vi "Query Active DUT Band Restrictions.vi"(8 "error in (no error)":errorcluster, 9 "Band Number (1)":i32=1, 10 "Band Type (LTE)":i32(ring) items=["LTE", "New Radio"], 11 "VISA resource name":refnum<visa-resource-name>) -> (0 "error out":errorcluster, 1 "RX":i32, 2 "TX":i32, 3 "VISA resource name out":refnum<visa-resource-name>)   [LabVIEW 2020, in "Rohde&Schwarz CMXP Base.lvlib"]
doc: "Queries restrictions for a frequency band assigned to connectors of the active DUT.\n\nAttribute:\n-\n\nRemote-control command:\n[CONFigure:]DUT:BAND:RESTrictions"
uses:
  <instrlib>/Rohde&Schwarz CMXP Base/Rohde&Schwarz CMXP Base.lvlib
  <instrlib>/Rohde&Schwarz CMXP Base/Private/rsidr_core.llb/rsidr_core.lvlib
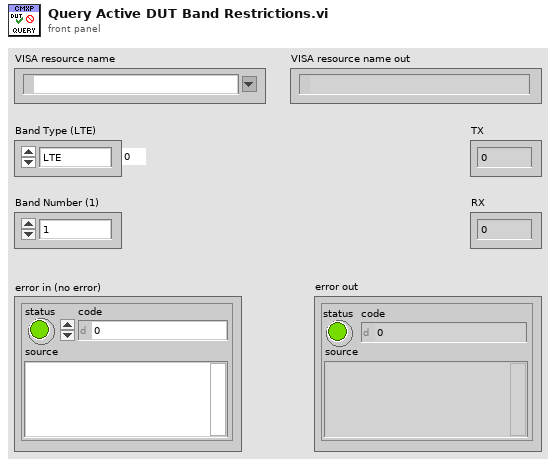
[diagram p1: front panel]
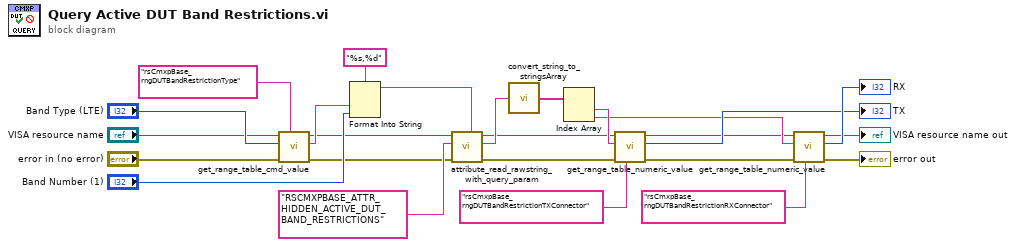
[diagram p0: block diagram]
diagram:
  n1 = call <instrlib>:"get_range_table_cmd_value.vi"("Range Table ID in"="rsCmxpBase_rngDUTBandRestrictionType", "error in"="error in (no error)", "Input Int32 value"="Band Type (LTE)", "VISA resource name"="VISA resource name") -> ("error out"=w8:errorcluster, "Cmd value out"=w11:string, "VISA resource name out"=w7:refnum<visa-resource-name>)  [unwired: 5 in]
  n2 = Format Into String(format string="%s,%d", w11, "Band Number (1)") -> (resulting string=w21:string)  [unwired: 2 in, 1 out]
  n3 = call <instrlib>:"attribute_read_rawstring_with_query_param.vi"("Query Parameter (None)"=w21, "error in"=w8, "Attribute ID"="RSCMXPBASE_ATTR_HIDDEN_ACTIVE_DUT_BAND_RESTRICTIONS", "VISA resource name"=w7) -> ("error out"=w6:errorcluster, "RawString out"=w12:string, "VISA resource name out"=w5:refnum<visa-resource-name>)  [unwired: 5 in]
  n4 = call <instrlib>:"convert_string_to_stringsArray.vi"("String in"=w12) -> ("string array out"=w20:string[])  [unwired: 3 in, 1 out]
  n5 = Index Array(array=w20) -> (element #1=w19:string, element #2=w13:string)  [unwired: 2 in]
  n6 = call <instrlib>:"get_range_table_numeric_value.vi"("Range Table ID in"="rsCmxpBase_rngDUTBandRestrictionTXConnector", "error in"=w6, "String Value"=w19, "VISA resource name"=w5) -> ("error out"=w4:errorcluster, "I32 output"=→"TX":i32, "VISA resource name out"=w3:refnum<visa-resource-name>)  [unwired: 5 in]
  n7 = call <instrlib>:"get_range_table_numeric_value.vi"("Range Table ID in"="rsCmxpBase_rngDUTBandRestrictionRXConnector", "error in"=w4, "String Value"=w13, "VISA resource name"=w3) -> ("error out"=→"error out":errorcluster, "I32 output"=→"RX":i32, "VISA resource name out"=→"VISA resource name out":refnum<visa-resource-name>)  [unwired: 5 in]
